vi "outputs.vi"() -> ()   [LabVIEW 2019]
doc: "This global variable contains current robot state information and actuator setpoints."
panel:
  out "Current_Driver_Profile_Setpoints":dbl[](array[numeric])
  out "Selected_Shooter_Setpoint_Value (rpm)":dbl
  out "Magazine_On":bool
  out "Magazine_Power":dbl
  out "Climber_Climbing":bool
  out "PTO":bool
  out "Climber_Pin":bool
  out "Climber_Power":dbl
  out "Disallowed_Shooter_States":bool[](array[boolean])
  out "Shooter_Needs_Power":bool
  out "Shooter_Spinning":bool
  out "Kicker_Goal_Speed (rpm)":dbl
  out "Shooter_Ready":bool
  out "Cowl_State":string
  out "Cowl_Piston":bool
  out "Out_Of_Range":bool
  out "Confirmed_Shooter_States":bool[](array[boolean])
  out "Shooter_Firing":bool
  out "Shooter_Goal_Speed (rpm)":dbl
  out "LED_Colors":u32[](array[colorbox])
  out "LimeLight_LED_Mode":enum16{"Pipeline Setting", "Off", "Blink", "On"}(ring)=enum."Off"
  out "LimeLight_Pipeline":T1(ring)
  out "Force_Low_Gear":bool
  out "Swerve_2_High_Gear_Requested":bool
  out "Swerve_1_High_Gear_Requested":bool
  out "Swerve_3_High_Gear_Requested":bool
  out "Swerve_0_High_Gear_Requested":bool
  out "Swerve_2_Drive_Flip":bool
  out "Swerve_1_Drive_Flip":bool
  out "Swerve_3_Drive_Flip":bool
  out "Swerve_0_Drive_Flip":bool
  out "Swerve_3_Azimuth_Goal (deg)":dbl
  out "Swerve_1_Azimuth_Goal (deg)":dbl
  out "Swerve_2_Azimuth_Goal (deg)":dbl
  out "Swerve_0_Azimuth_Goal (deg)":dbl
  out "Diverting_Power_LEDS":bool
  out "Swerve_Rotation_Command":dbl
  out "Disallowed_Master_States":bool[](array[boolean])
  out "Drive_Mode":T2(ring)
  out "Intake_Deployed":bool
  out "Diverting_Power_Compressor":bool
  out "Intake_On":bool
  out "Intake_Power":dbl
  out "Field_Oriented":bool
  out "Confirmed_Master_States":bool[](array[boolean])
  out "Boost_Drive_Current_Limit":bool
  out "Swerve_3_Azimuth_Error (deg)":dbl
  out "Swerve_1_Azimuth_Error (deg)":dbl
  out "Swerve_2_Azimuth_Error (deg)":dbl
  out "Swerve_0_Azimuth_Error (deg)":dbl
  out "Swerve_3_Drive_Command":dbl
  out "Swerve_1_Drive_Command":dbl
  out "Swerve_2_Drive_Command":dbl
  out "Swerve_0_Drive_Command":dbl
  # "--master state controller--"
  # "--drivebase subsystem--"
  # "--ball handling subsystem--"
  # "--power management--"
  # "--LL control--"
  # "--LEDs--"
  # "--climber subsystem--"
  # "--shooter subsystem--"
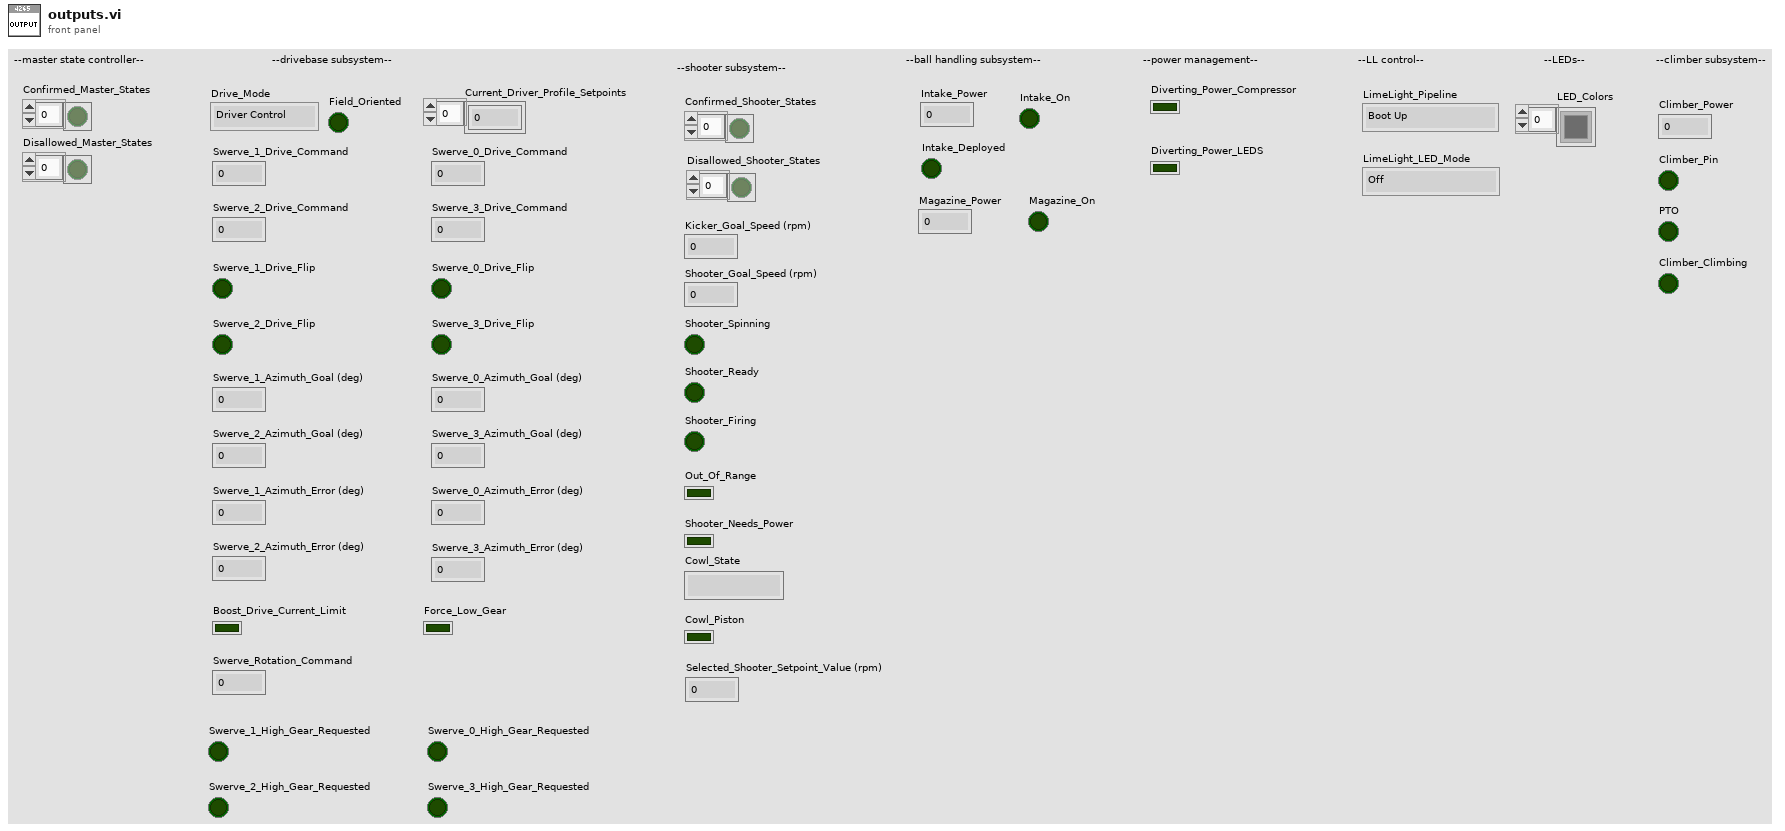
[diagram p1: front panel]
types:
  T1 = enum16{"Boot Up", "Camera Override", "Power Port", "Ball Tracking"}
  T2 = enum16{"Driver Control", "Auto Targeting", "Feeder Station"}
diagram:
